vi "Update_twaveformsdata_example_Core.vi"() -> ()   [LabVIEW 2011]
uses:
  <vilib>/addons/database/Connection.llb/DB Tools Open Connec (String).vi
  <vilib>/Analysis/1siggen.llb/Ramp Pattern by Samples.vi
  <vilib>/addons/database/_DB Variant To Data/Database Variant To Data.xnode
  <vilib>/addons/database/NI_Database_API.lvlib
  <vilib>/Analysis/NI_AALBase.lvlib
panel:
  out "subarray":dbl[](graph)
  out "data":dbl[][](graph)
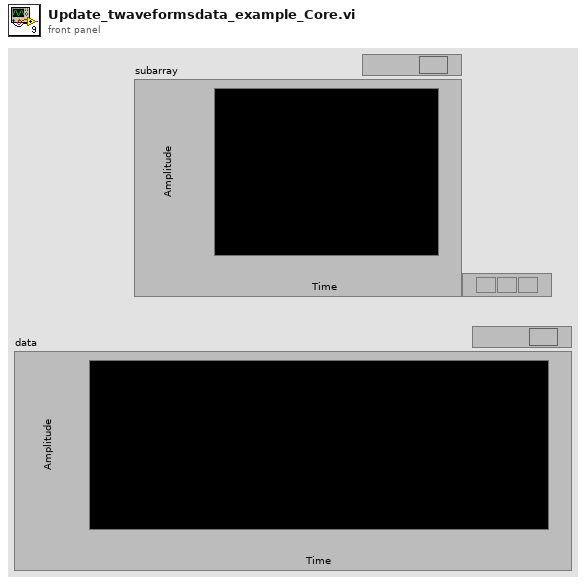
[diagram p1: front panel]
types:
  T1 = typedef "NI_Database_API.lvlib/Conn ObjectReference.ctl" = refnum<k1>
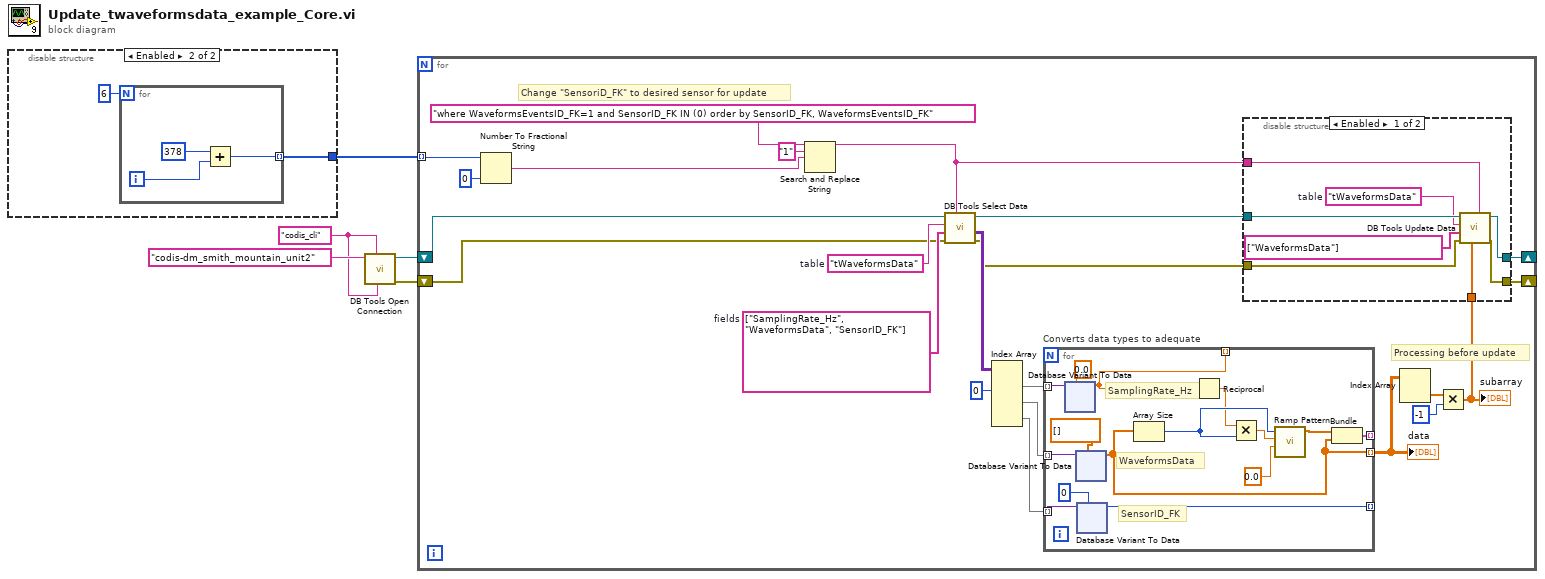
[diagram p0: block diagram]
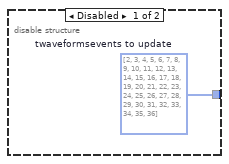
[diagram p2: hidden frame]
diagram:
  w3 = "codis_cli" ("userID")
  n1 = disable-structure shown="Enabled" {
    disable-tunnel: [w6 w8] -> w5
    frame Disabled {
      w6 = u32[] [2, 3, 4, 5, 6, 7, 8, 9, 10, 11, 12, 13, 14, 15, 16, 17, 18, 19, 20, 21, 22, 23, 24, 25, 26, 27, 28, 29, 30, 31, 32, 33, 34, 35, 36]  # twaveformsevents to update
    }
    frame Enabled {
      n2 = for {
        N: 6 -> [_]
        tunnel: [w9] -> w8 mode=indexing
        i -> [w11]
        n3 = Add(x=378, y=w11) -> (x+y=w9:i32)
      }
    }
  }
  n4 = call-poly <vilib>:"DB Tools Open Connection.vi"("password"=w3, "userID"=w3, "connection information"="codis-dm_smith_mountain_unit2" ("userID")) -> ("error out"=w1:errorcluster, "connection reference"=w2:T1)  [unwired: 5 in]
  n5 = for {
    tunnel: w5 -> [w22] mode=indexing
    shift-right: [w14] -> _
    shift-left: w2 -> [w16]
    shift-right: [w12] -> _
    shift-left: w1 -> [w15]
    w33 = string[] ["SamplingRate_Hz", "WaveformsData", "SensorID_FK"]  # fields
    w34 = "tWaveformsData"  # table
    # "Processing before update"
    # "Change \"SensoriD_FK\" to desired sensor for update"
    n6 = Number To Fractional String(number=w22, precision (6)=i16 0) -> (F-format string=w18:string)  [unwired: 2 in]
    n7 = Search and Replace String(input string="where WaveformsEventsID_FK=1 and SensorID_FK IN (0) order by SensorID_FK, WaveformsEventsID_FK", search string="1", replace string=w18) -> (result string=w17:string)  [unwired: 5 in, 3 out]
    n8 = call <vilib>:"DB Tools Select Data.vi"("condition"=w17, "error in (no error)"=w15, "columns"=w33, "table"=w34, "connection reference"=w16) -> ("error out"=w13:errorcluster, "data"=w28:variant[][], "connection reference out"=w27:T1)  [unwired: 1 in]
    n9 = Index Array(array=w28, index (col) #1=0 ("disabled index (col)")) -> (element #1=w31:variant[], element #2=w30:variant[], element #3=w29:variant[])  [unwired: 5 in]
    n10 = for "Converts data types to adequate" {
      tunnel: w31 -> [w57] mode=indexing
      tunnel: w30 -> [w56] mode=indexing
      tunnel: [w49] -> _ mode=indexing
      tunnel: w29 -> [w48] mode=indexing
      tunnel: [w46] -> _ mode=indexing
      tunnel: [w44] -> _ mode=indexing
      tunnel: [w43] -> w26 mode=indexing
      # "SensorID_FK"
      # "WaveformsData"
      # "SamplingRate_Hz"
      n11 = xnode "Database Variant To Data"("database variant"=w57, "type"=0.0) -> ("data"=w44:dbl)  [unwired: 1 in, 1 out]
      n12 = xnode "Database Variant To Data"("database variant"=w56, "type"=dbl[] []) -> ("data"=w43:dbl[])  [unwired: 1 in, 1 out]
      n13 = xnode "Database Variant To Data"("database variant"=w48, "type"=u8 0) -> ("data"=w46:u8)  [unwired: 1 in, 1 out]
      n14 = Array Size(array=w43) -> (size(s)=w52:i32)
      n15 = Reciprocal(x=w44) -> (1/x=w45:dbl)
      n16 = Multiply(x=w45, y=w52) -> (x*y=w51:dbl)
      n17 = call-poly <vilib>:"Ramp Pattern.vi"("start"=0.0, "end"=w51, "samples"=w52) -> ("Ramp Pattern"=w50:dbl[])  [unwired: 7 in, 1 out]
      n18 = Bundle("Ramp Pattern"=w50, "data"=w43) -> (w49:cluster{"Ramp Pattern":dbl[], "data":dbl[]})  [unwired: 1 in]
    }
    "data" <- w26
    n19 = Index Array(array=w26) -> (element=w25:dbl[])  [unwired: 2 in]
    n20 = Multiply(x=w25, y=-1) -> (x*y=w24:dbl[])
    "subarray" <- w24
    n21 = disable-structure shown="Enabled" {
      disable-tunnel: w27 -> [w42 _]
      disable-tunnel: w17 -> [w39 _]
      disable-tunnel: w24 -> [w38 _]
      disable-tunnel: [w37 _] -> w14
      disable-tunnel: w13 -> [w36 _]
      disable-tunnel: [w35 _] -> w12
      frame Enabled {
        w40 = "tWaveformsData"  # table
        n22 = call <vilib>:"DB Tools Update Data.vi"("condition"=w39, "data"=w38, "error in (no error)"=w36, "columns"=string[] ["WaveformsData"], "table"=w40, "connection reference"=w42) -> ("error out"=w35:errorcluster, "connection reference out"=w37:T1)  [unwired: 4 in]
      }
      frame Disabled {
      }
    }
  }
